vi "Save Constants Info next to LV Project.vi"(10 "Constant Info Results Str":string[][](array[string]), 11 "Project Path":path) -> ()   [LabVIEW 2020, in "ConstantErrorsMaker.lvlib"]
uses:
  ConstantErrorsMaker.lvlib
  <vilib>/Utility/file.llb/Write Delimited Spreadsheet (string).vi
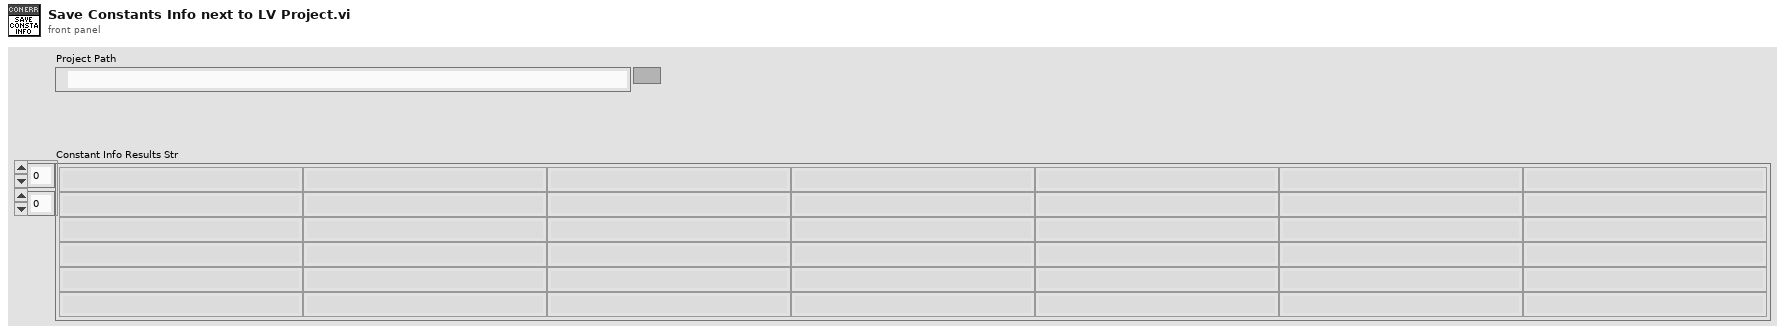
[diagram p1: front panel]
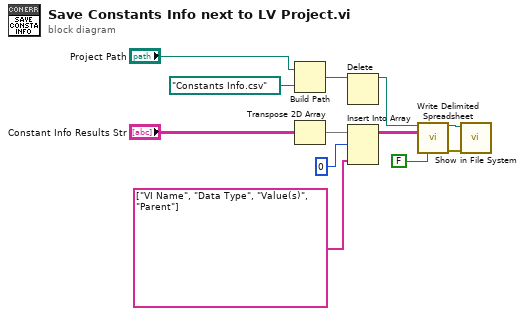
[diagram p0: block diagram]
diagram:
  n1 = Build Path(base path="Project Path", name or relative path=path "Constants Info.csv") -> (appended path=w7:path)
  n2 = Transpose 2D Array(2D array="Constant Info Results Str") -> (transposed array=w1:string[][])
  n3 = Delete(path (use dialog)=w7) -> (deleted path=w8:path)  [unwired: 4 in, 2 out]
  n4 = Insert Into Array(array=w1, index (row)=0, new element=string[] ["VI Name", "Data Type", "Value(s)", "Parent"]) -> (w10:string[][])  [unwired: 1 in]
  n5 = call-poly <vilib>:"Write Delimited Spreadsheet.vi"("file path (dialog if empty)"=w8, "2D data"=w10, "transpose? (no:F)"=FALSE) -> ("new file path (Not A Path if cancelled)"=w5:path, "error out"=w12:errorcluster)  [unwired: 11 in]
  n6 = call <vilib>:"Show in File System.vi"("error in (no error)"=w12, "file or directory path"=w5) -> ()  [unwired: 9 in, 1 out]
